vi "Two Color Cal Find Focus.vi"(0 "Camera Notifier Name":string, 11 "Z Stage Notifier Name":string) -> (4 "Camera Notifier (Dup)":string)   [LabVIEW 2016]
uses:
  Device Library/Stages/Stages Controls/Stage Actions.ctl
  Device Library/Cameras/Camera Controls/Generic Camera Actions.ctl
  <vilib>/Analysis/NI_AALPro.lvlib
  <vilib>/Analysis/6fits.llb/Curve Fitting Criteria.ctl
  <vilib>/gmath/NI_Gmath.lvlib
panel:
  out "Focus Position":dbl
  out "Fitted Width vs Position":cluster{dbl[], dbl[]}[](graph)
  out "Step Number":i32
  out "Bead Image":T1(plugin-control)
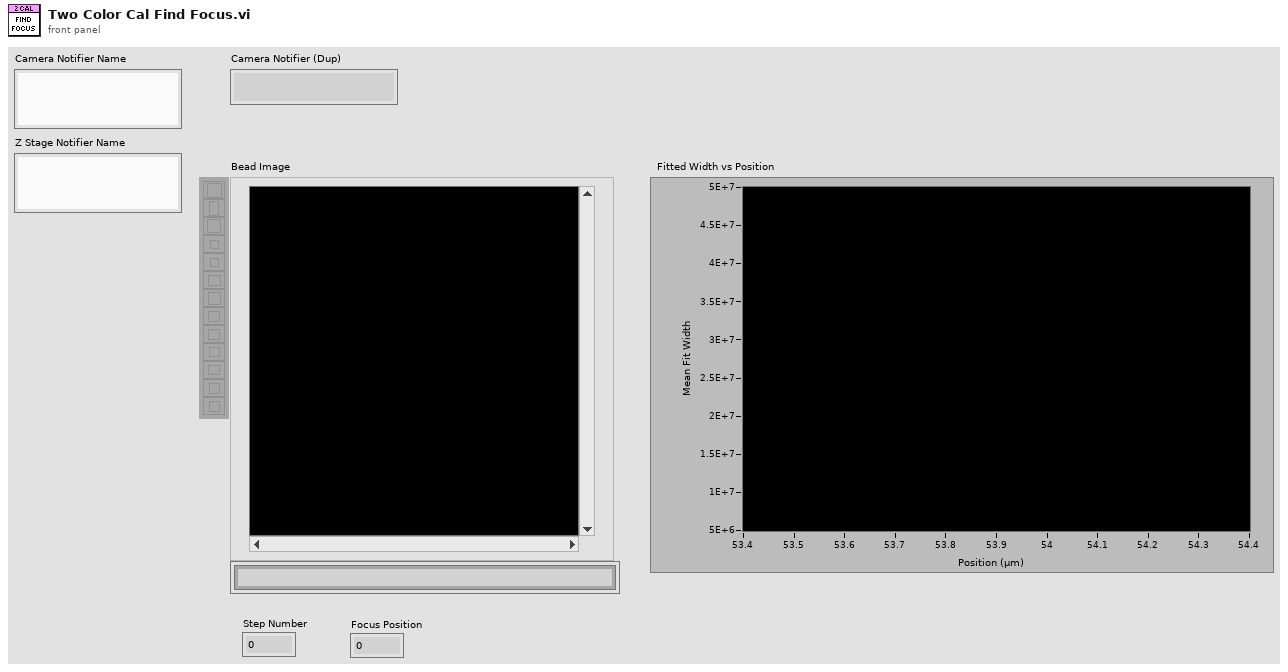
[diagram p1: front panel]
types:
  T1 = typedef "IMAQ Image.ctl" = refnum<image>
  T2 = typedef "Stage Actions.ctl" = enum16{"Get Position", "MVR", "MOVE", "HALT", "ONTARGET", "ERROR", "REFERENCE", "INIT", "VELOCITY", "STATUS", "EXIT", "HOME", "ZEROPOS", "NANOPOS", "ANALOG", "QUIT"}
  T3 = typedef "Generic Camera Actions.ctl" = enum16{"Status", "Live Preview", "Capture", "Abort", "Set Exposure Time (s)", "Get Exposure Time (s)", "Record Settings", "Set ROI", "Get ROI", "Defect Correction On/Off", "Cooler On/Off", "Fan On/Off", "Quti"}
  T4 = cluster{"Global Rectangle":i32[], "Contours":cluster{"Contour Type":u32, "ROI Type":u32, "Points":i32[]}[]}
  T5 = typedef "2D Gaussian - Best Fit Parameters.ctl" = cluster{"Amplitude":dbl, "X Position":dbl, "Y Position":dbl, "X Width":dbl, "Y Width":dbl, "Offset":dbl}
  T6 = enum16{"Linear", "Polynomial", "Exponential", "Power"}
  T7 = typedef "NI_AALPro.lvlib/Curve Fitting Criteria.ctl" = u16
  T8 = cluster{"X Values Out":dbl[], "Y Values Out":dbl[]}
  T9 = cluster{"X Values Out":dbl[], "Y Values Out":dbl[]}[]
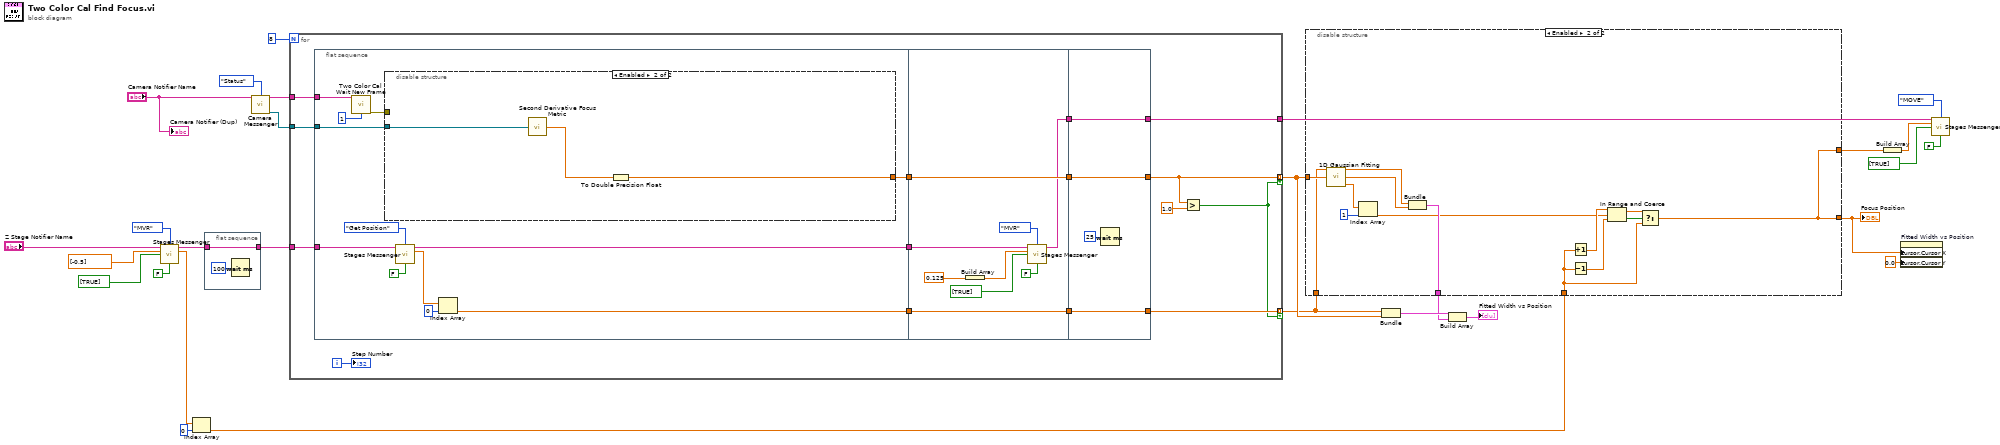
[diagram p0: block diagram]
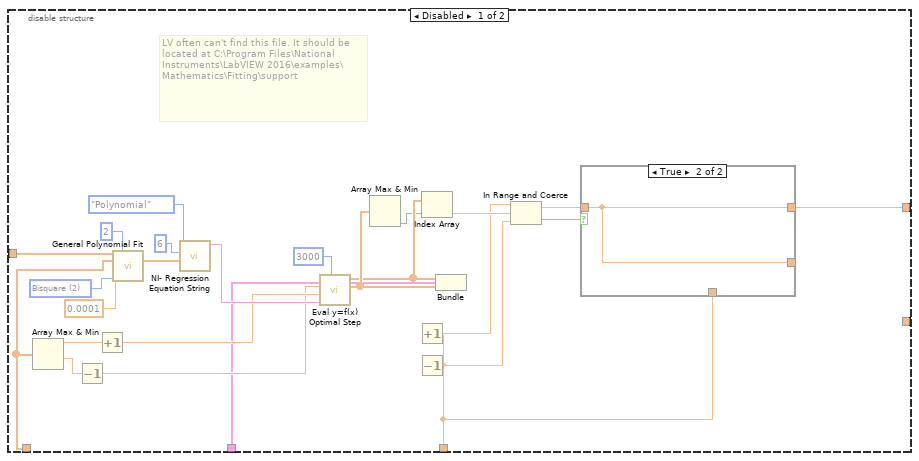
[diagram p2: hidden frame]
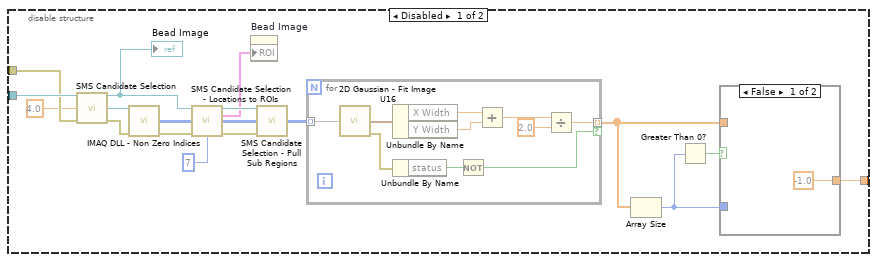
[diagram p4: hidden frame]
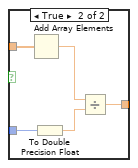
[diagram p5: hidden frame]
diagram:
  n1 = call "Stages Messenger.vi"("Stage Notifier Name"="Z Stage Notifier Name", "Actions"=Stage_Actions."MVR", "Setpoint"=dbl[] [-0.5], "Axis"=bool[] [TRUE], "Exit While Busy?"=FALSE) -> ("Stage Notifier Name (Dup)"=w23:string, "Positions"=w14:dbl[])  [unwired: 7 in, 2 out]
  n2 = Index Array(array=w14, index=0) -> (element=w10:dbl)
  n3 = flat-sequence {
    tunnel: w23 -> [w29]
    tunnel: [w29] -> w22
    frame #0 {
      n4 = Wait (ms)(milliseconds to wait=u32 100) -> ()  [unwired: 1 out]
    }
  }
  n5 = call "Camera Messenger.vi"("Notifier Name"="Camera Notifier Name", "General Camera Actions"=Generic_Camera_Actions."Status") -> ("Notifier Name Dup"=w18:string, "Image Ref"=w17:T1)  [unwired: 8 in, 4 out]
  n6 = for {
    N: 8 -> [_]
    tunnel: w22 -> [w43]
    tunnel: w18 -> [w45]
    tunnel: w17 -> [w44]
    tunnel: [w38] -> w15 mode=indexing if=w31
    tunnel: [w33] -> w16 mode=indexing if=w31
    tunnel: [w34] -> w12
    i -> [w41]
    n7 = flat-sequence {
      tunnel: w45 -> [w57]
      tunnel: w44 -> [w56]
      tunnel: w43 -> [w51]
      tunnel: [w48] -> w42
      tunnel: [w47] -> w39
      tunnel: [w46] -> w36
      tunnel: w42 -> [w98]
      tunnel: [w97] -> w40
      tunnel: w39 -> [w97]
      tunnel: [w96] -> w37
      tunnel: w36 -> [w96]
      tunnel: [w95] -> w35
      tunnel: [w106] -> w38
      tunnel: w40 -> [w106]
      tunnel: w37 -> [w105]
      tunnel: [w105] -> w33
      tunnel: [w104] -> w34
      tunnel: w35 -> [w104]
      frame #0 {
        n8 = call "Two Color Cal Wait New Frame.vi"("Notifier Name"=w57, "Frames to Wait"=u32 1) -> ("Error Out"=w54:errorcluster)  [unwired: 13 in]
        n9 = disable-structure shown="Enabled" {
          disable-tunnel: w56 -> [w67 w94]
          disable-tunnel: w54 -> [w66 _]
          disable-tunnel: [w61 w92] -> w46
          frame Disabled {
            n10 = call "SMS Candidate Selection.vi"("Image Ref (U16)"=w67, "Blink Sensitivity"=sgl 4.0, "Error In"=w66) -> ("Image Ref (U16) - Dup"=w64:T1, "Cadidate Image Ref"=w75:T1, "Error Out"=w74:errorcluster)  [unwired: 10 in]
            "Bead Image" <- w64
            n11 = call "IMAQ DLL - Non Zero Indices.vi"("IMAQ Ref"=w75, "Error In"=w74) -> ("Row Column Indices"=w73:i32[][], "Error Out"=w72:errorcluster)  [unwired: 10 in, 2 out]
            n12 = call "SMS Candidate Selection - Locations to ROIs.vi"("Image Ref"=w64, "Row Column Indices"=w73, "Error"=w72, "Box Half Size"=u8 7) -> ("Image Ref (DUP)"=w71:T1, "Image ROIs"=w65:T4, "ROI Coordinates (Left, Top, Right, Bottom)"=w70:i32[][], "Error Out"=w69:errorcluster)  [unwired: 8 in]
            n13 = property on="Bead Image" class="ImageControl"("ROI"=w65) -> ()  [unwired: 2 in, 2 out]
            n14 = call "SMS Candidate Selection - Pull Sub Regions.vi"("Image Ref"=w71, "ROI Coordinates"=w70, "Error"=w69) -> ("ROIs"=w62:u16[][][])  [unwired: 10 in, 2 out]
            n15 = for {
              tunnel: w62 -> [w91] mode=indexing
              tunnel: [w85] -> w60 mode=indexing if=w82
              n16 = call "2D Gaussian - Fit Image U16.vi"("Image In (U16)"=w91) -> ("Best Fit Params"=w90:T5, "Error Out"=w84:errorcluster)  [unwired: 13 in]
              n17 = Unbundle By Name(w90) -> ("X Width"=w89:dbl, "Y Width"=w88:dbl)
              n18 = Unbundle By Name(w84) -> ("status"=w83:bool)
              n19 = Not(x=w83) -> (.not. x?=w82:bool)
              n20 = Add(x=w89, y=w88) -> (x+y=w87:dbl)
              n21 = Divide(x=w87, y=2.0) -> (x/y=w85:dbl)
            }
            n22 = Array Size(array=w60) -> (size(s)=w58:i32)
            n23 = Greater Than 0?(x=w58) -> (x > 0?=w59:bool)
            n24 = case shown="False" w59 {
              tunnel: [-1.0 w80] -> w61
              tunnel: w60 -> [_ w79]
              tunnel: w58 -> [_ w78]
              frame False {
              }
              frame True {
                n25 = Add Array Elements(numeric array=w79) -> (sum=w77:dbl)
                n26 = To Double Precision Float(number=w78) -> (double precision float=w81:dbl)
                n27 = Divide(x=w77, y=w81) -> (x/y=w80:dbl)
              }
            }
          }
          frame Enabled {
            n28 = call "Second Derivative Focus Metric.vi"("Image Ref (U16)"=w94) -> ("LAP_VAR"=w93:sgl)  [unwired: 14 in]
            n29 = To Double Precision Float(number=w93) -> (double precision float=w92:dbl)
          }
        }
        n30 = call "Stages Messenger.vi"("Stage Notifier Name"=w51, "Actions"=Stage_Actions."Get Position", "Exit While Busy?"=FALSE) -> ("Stage Notifier Name (Dup)"=w48:string, "Positions"=w50:dbl[])  [unwired: 9 in, 2 out]
        n31 = Index Array(array=w50, index=0) -> (element=w47:dbl)
      }
      frame #1 {
        n32 = Build Array(0.125 ("Z Step Size")) -> (w103:dbl[])
        n33 = call "Stages Messenger.vi"("Stage Notifier Name"=w98, "Actions"=Stage_Actions."MVR", "Setpoint"=w103, "Axis"=bool[] [TRUE], "Exit While Busy?"=FALSE) -> ("Stage Notifier Name (Dup)"=w95:string)  [unwired: 7 in, 3 out]
      }
      frame #2 {
        n34 = Wait (ms)(milliseconds to wait=u32 25) -> ()  [unwired: 1 out]
      }
    }
    n35 = Greater?(x=w33, y=1.0) -> (0:w31:bool)
    "Step Number" <- w41
  }
  n36 = disable-structure shown="Enabled" {
    disable-tunnel: w16 -> [w125 w148]
    disable-tunnel: w15 -> [w124 w147]
    disable-tunnel: [w110 w135] -> w11
    disable-tunnel: w10 -> [w109 w136]
    disable-tunnel: [w108 w144] -> w7
    disable-tunnel: [_ w135] -> w5
    frame Disabled {
      w132 = T7 2 items=["Least Square", "Least Absolute Residual", "Bisquare"] ("method")
      # "LV often can't find this file. It should be located at C:\\Program Files\\National Instruments\\LabVIEW 2016\\examples\\Mathematics\\Fitting\\support"
      n37 = Array Max & Min(array=w124) -> (max value=w119:dbl, min value=w120:dbl)  [unwired: 2 out]
      n38 = Decrement(x=w120) -> (x-1=w117:dbl)
      n39 = Increment(x=w119) -> (x+1=w118:dbl)
      n40 = call <vilib>:"General Polynomial Fit.vi"("Y"=w125, "polynomial order"=2, "X"=w124, "tolerance"=0.0001, "method"=w132) -> ("Polynomial Coefficients"=w129:dbl[])  [unwired: 7 in, 3 out]
      n41 = call "NI- Regression Equation String.vi"("coefficients"=w129, "precision"=6, "fit type"=T6."Polynomial") -> ("Formula"=w127:string)  [unwired: 8 in]
      n42 = call <vilib>:"Eval y=f(x) Optimal Step.vi"("number of points"=u32 3000, "formula"=w127, "end"=w118, "start"=w117) -> ("Y Values"=w123:dbl[], "X Values"=w122:dbl[])  [unwired: 1 in, 2 out]
      n43 = Array Max & Min(array=w123) -> (min index (indices)=w121:i32)  [unwired: 3 out]
      n44 = Increment(x=w109) -> (x+1=w112:dbl)
      n45 = Decrement(x=w109) -> (x-1=w111:dbl)
      n46 = Index Array(array=w122, index=w121) -> (element=w115:dbl)
      n47 = Bundle("X Values"=w122, "Y Values"=w123) -> (w108:cluster{"X Values":dbl[], "Y Values":dbl[]})  [unwired: 1 in]
      n48 = In Range and Coerce(upper limit=w112, x=w115, lower limit=w111) -> (coerced(x)=w114:dbl, In Range?=w113:bool)
      n49 = case shown="True" w113 {
        tunnel: w114 -> [_ w134]
        tunnel: [w133 w134] -> _
        tunnel: [w133 w134] -> w110
        tunnel: w109 -> [w133 _]
        frame False {
        }
        frame True {
        }
      }
    }
    frame Enabled {
      n50 = call "1D Gaussian Fitting.vi"("X Values"=w147, "Y Values"=w148) -> ("X Values Out"=w146:dbl[], "Y Values Out"=w145:dbl[], "Best Fit Parameters"=w143:dbl[])  [unwired: 11 in]
      n51 = Index Array(array=w143, index=1) -> (element=w139:dbl)
      n52 = Bundle("X Values Out"=w146, "Y Values Out"=w145) -> (w144:T8)  [unwired: 1 in]
      n53 = Increment(x=w136) -> (x+1=w141:dbl)
      n54 = Decrement(x=w136) -> (x-1=w140:dbl)
      n55 = In Range and Coerce(upper limit=w141, x=w139, lower limit=w140) -> (coerced(x)=w137:dbl, In Range?=w138:bool)
      n56 = Select(t=w137, s=w138, f=w136) -> (s? t:f=w135:dbl)
    }
  }
  "Focus Position" <- w5
  n57 = Bundle(w15, w16) -> (w9:cluster{dbl[], dbl[]})  [unwired: 1 in]
  n58 = Build Array(w9, w7) -> (→"Fitted Width vs Position":T9)
  n59 = Build Array(w11) -> (w4:dbl[])
  n60 = property on="Fitted Width vs Position" class="XYGraph (strict)"("Cursor.Cursor X"=w5, "Cursor.Cursor Y"=0.0 ("Cursor.Cursor Position:Cursor Y")) -> ()  [unwired: 2 in, 2 out]
  n61 = call "Stages Messenger.vi"("Stage Notifier Name"=w12, "Actions"=Stage_Actions."MOVE", "Setpoint"=w4, "Axis"=bool[] [TRUE], "Exit While Busy?"=FALSE) -> ()  [unwired: 7 in, 4 out]
  "Camera Notifier (Dup)" <- "Camera Notifier Name"
